vi "HTTP String.vi"(8 "Error In":errorcluster, 11 "String in":string) -> (0 "Error Out":errorcluster, 3 "String out":string)   [LabVIEW 2011, in "LMH-Toolbox.lvlib" / "LMH-Documentation.lvlib"]
uses:
  LMH-Documentation.lvlib
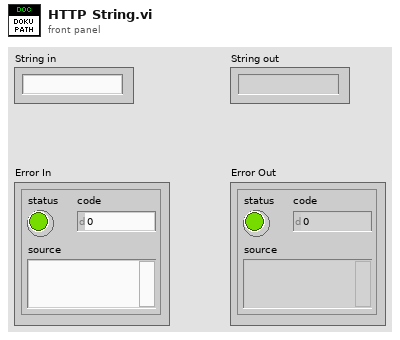
[diagram p1: front panel]
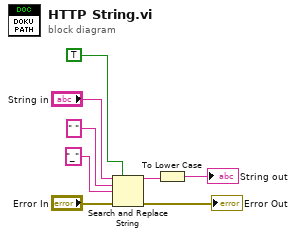
[diagram p0: block diagram]
diagram:
  n1 = Search and Replace String(replace all?=TRUE ("replace all? (F)"), input string="String in", search string=" ", replace string="_" ("replace string (\"\")"), error in="Error In") -> (result string=w2:string, error out=→"Error Out":errorcluster)  [unwired: 3 in, 2 out]
  n2 = To Lower Case(string=w2) -> (all lower case string=→"String out":string)
